vi "Check test status.vi"(10 "register values":u16[](array[numeric]), 11 "System data in":T1) -> (3 "System data out":T1)   [LabVIEW 2023]
uses:
  System Data.ctl
  <vilib>/NI/Modbus Library/API/Master/Modbus Master.lvclass
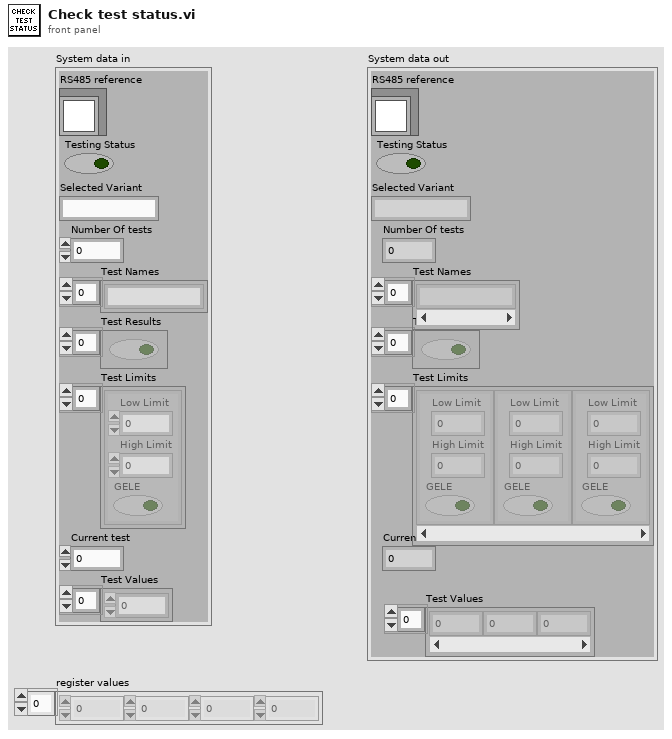
[diagram p1: front panel]
types:
  T1 = typedef "System Data.ctl" = cluster{"RS485 reference":refnum<class "Modbus Master.lvclass">, "Testing Status":bool, "Selected Variant":string, "Number Of tests":i32, "Test Names":string[], "Test Results":bool[], "Test Limits":cluster{"Low Limit":dbl, "High Limit":dbl, "GELE":bool}[], "Current test":i32, "Test Values":dbl[]}
  T2 = cluster{"Low Limit":dbl, "High Limit":dbl, "GELE":bool}[]
  T3 = cluster{"Low Limit":dbl, "High Limit":dbl, "GELE":bool}
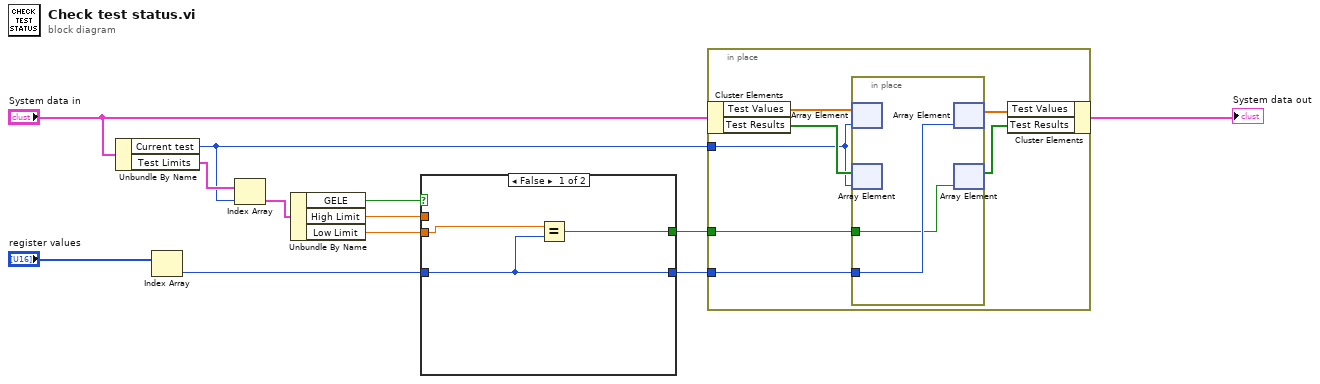
[diagram p0: block diagram]
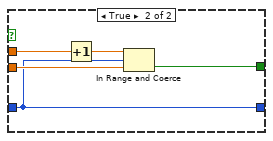
[diagram p2: hidden frame]
diagram:
  n1 = Unbundle By Name("System data in") -> ("Current test"=w9:i32, "Test Limits"=w10:T2)
  n2 = Index Array(array="register values") -> (element=w4:u16)  [unwired: 1 in]
  n3 = Index Array(array=w10, index=w9) -> (element=w8:T3)
  n4 = Unbundle By Name(w8) -> ("GELE"=w7:bool, "High Limit"=w6:dbl, "Low Limit"=w5:dbl)
  n5 = case shown="False" w7 {
    tunnel: w6 -> [_ w20]
    tunnel: w5 -> [w15 w19]
    tunnel: w4 -> [w13 w17]
    tunnel: [w14 w18] -> w2
    tunnel: [w13 w17] -> w3
    frame False {
      n6 = Equal?(x=w15, y=w13) -> (x = y?=w14:bool)
    }
    frame True {
      n7 = Increment(x=w20) -> (x+1=w16:dbl)
      n8 = In Range and Coerce(upper limit=w16, x=w17, lower limit=w19) -> (In Range?=w18:bool)  [unwired: 1 out]
    }
  }
  n9 = in-place {
    in-place-border: w9 -> [w23]
    in-place-border: w3 -> [w22]
    in-place-border: w2 -> [w21]
    n10 = in-place-cluster #1("System data in") -> ("Test Values"=w27:dbl[], "Test Results"=w26:bool[])
    n11 = in-place {
      in-place-border: w22 -> [w29]
      in-place-border: w21 -> [w28]
      n12 = in-place-array #2(w27, w23) -> ()  [unwired: 1 out]
      n13 = in-place-array #3(w26, w23) -> ()  [unwired: 1 out]
      n14 = in-place-array #2(w29) -> (w25:dbl[])  [unwired: 1 out]
      n15 = in-place-array #3(w28) -> (w24:bool[])  [unwired: 1 out]
    }
    n16 = in-place-cluster #1("Test Values"=w25, "Test Results"=w24) -> (→"System data out":T1)
  }
